vi "TCP_CC.vi"(4 "COMMAND":string, 5 "connection ID":refnum<k5>, 6 "error in (no error)":errorcluster, 7 "IP ADDRESS":string="192.168.0.2") -> (0 "number":u32, 1 "error out":errorcluster, 2 "connection ID out":refnum<k5>, 3 "Their Response:":string)   [LabVIEW 2013]
doc: "Demonstrates how to display an interactive send and receive message dialog for communication between TCP connections. It establishes a connection on the machine listed and the port specified. It then waits for you to input data into the Input Line string control and hit enter. Once you hit enter, the string you typed is sent to the port and passed to the TCP Communicator - Passive.vi where it is displayed on a string indicator.\n\nThe key difference between the Active and Passive VIs is that the Active VI establishes a connection, while the Passive VI waits for a connection to be established.\n\n<B>Note:</B> Requires the TCP Communicator - Passive.vi."
panel:
  out "x = y?":bool
  out "Boolean array":bool[](array[boolean])
  # "TS1 / TS2\nDISC / T0\nTEST\nDRIVE READY\nREG MODE\nDATA VETO\nSYNC MODE\nMOTOR TEMP\nDE BEARING TEMP\nBEARING TEMP\nDIRECTION\nEEP-SMP SYNC\nSPEED BIT 1\nSPEED BIT 2\nSPEED BIT 3\nSPEED BIT 4\nEEP\nCLK\nMP\nMP UNSYNC\nSMBBUS BUSY"
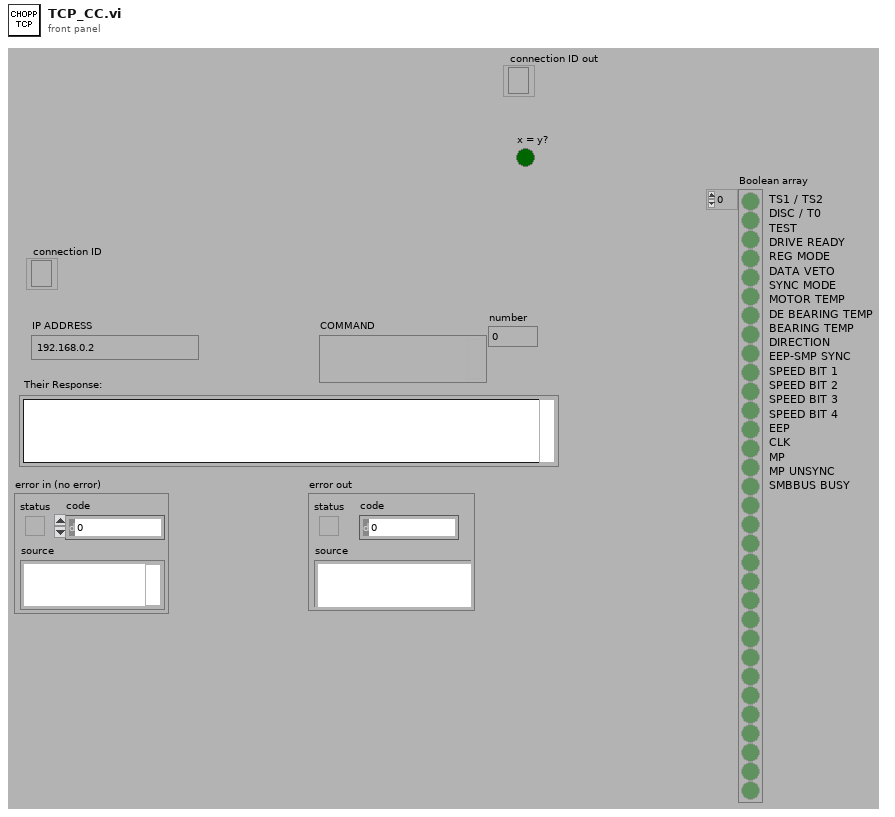
[diagram p1: front panel]
types:
  T1 = enum16{"Standard", "Buffered", "CRLF", "Immediate"}
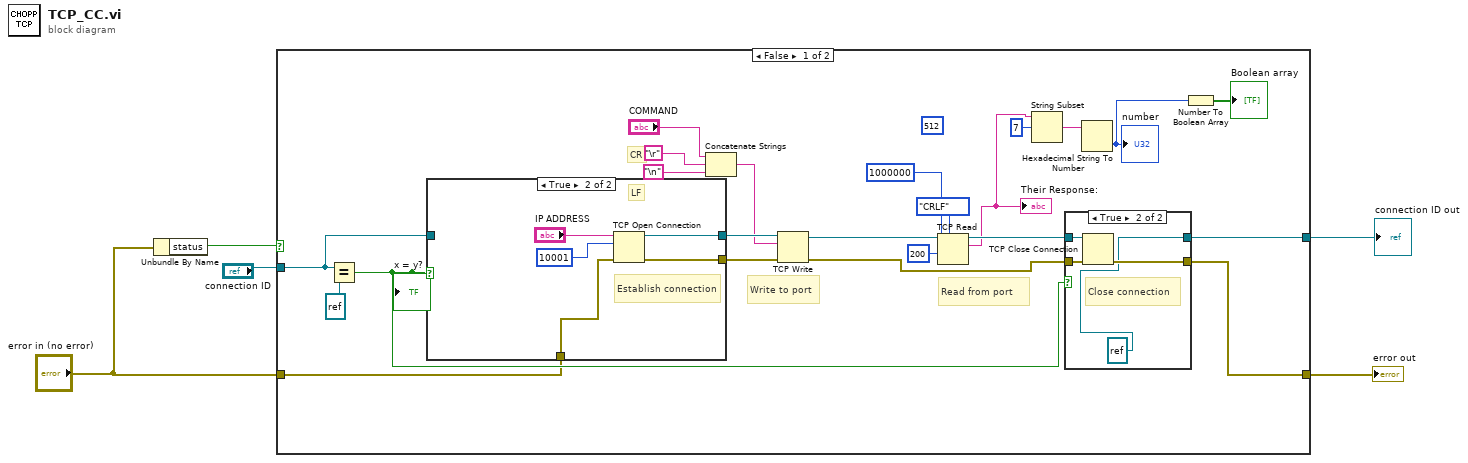
[diagram p0: block diagram]
diagram:
  n1 = Unbundle By Name("error in (no error)") -> ("status"=w3:bool)
  n2 = case shown="False" w3 {
    tunnel: "connection ID" -> [w14 w43]
    tunnel: [w13 w43] -> w4
    tunnel: "error in (no error)" -> [w7 w42]
    tunnel: [w6 w42] -> w1
    frame False {
      (unwired) 512
      # "Read from port"
      # "Write to port"
      # "CR"
      n3 = Equal?(x=w14, y=refnum<k5> refnum) -> (x = y?=w8:bool)
      "x = y?" <- w8
      n4 = case shown="True" w8 {
        tunnel: [w35 w40] -> w28
        tunnel: [w36 w39] -> w27
        tunnel: w14 -> [w36 _]
        tunnel: w7 -> [w35 w37]
        frame False {
        }
        frame True {
          # "LF"
          # "Establish connection"
          n5 = TCP Open Connection(address="IP ADDRESS", remote port or service name=u16 10001 ("remote port"), error in (no error)=w37) -> (connection ID=w39:refnum<k5>, error out=w40:errorcluster)  [unwired: 2 in]
        }
      }
      n6 = Concatenate Strings("COMMAND", "\r", "\n") -> (w23:string)
      n7 = TCP Write(connection ID=w27, data in=w23, error in (no error)=w28) -> (connection ID out=w11:refnum<k5>, error out=w21:errorcluster)  [unwired: 1 in, 1 out]
      n8 = TCP Read(connection ID=w11, bytes to read=1000000, 7:T1."CRLF" ("mode (standard)"), 9:200) -> (connection ID out=w26:refnum<k5>, data out=w18:string)  [unwired: 1 in, 1 out]
      "Their Response:" <- w18
      n9 = String Subset(string=w18, offset (0)=7) -> (substring=w20:string)  [unwired: 1 in]
      n10 = case shown="True" w8 {
        tunnel: w26 -> [w29 w34]
        tunnel: [w30 w33] -> w6
        tunnel: w21 -> [w30 w32]
        tunnel: [w29 refnum<k5> refnum ("y")] -> w13
        frame False {
        }
        frame True {
          # "Close connection"
          n11 = TCP Close Connection(connection ID=w34, error in (no error)=w32) -> (error out=w33:errorcluster)  [unwired: 1 in, 1 out]
        }
      }
      n12 = Hexadecimal String To Number(string=w20) -> (number=w17:u32)  [unwired: 2 in, 1 out]
      "number" <- w17
      n13 = Number To Boolean Array(number=w17) -> (Boolean array=→"Boolean array":bool[])
    }
    frame True {
    }
  }
  "connection ID out" <- w4
  "error out" <- w1
